vi "TL_init.vi"(0 "Channel #":i32, 1 "TL array":dbl[][](array[numeric]), 3 "Queue cluser":T1, 5 "Mosaic cluster":cluster{dbl[], dbl[]}[](array[cluster]), 7 "N ROIs":i32, 9 "error in":errorcluster, 11 "Start acquisition":bool, 12 "XYGraph":refnum<vi>, 14 "Dt (s)":i32) -> (6 "Ready":bool, 15 "error out":errorcluster)   [LabVIEW 2015]
uses:
  CONTROLS/Q_DAQ_element.ctl
  CONTROLS/Q_camera_element.ctl
  CONTROLS/Q_ASI_stage_element.ctl
  CONTROLS/Q_MCL_piezo_element.ctl
  GLOBAL/Global_DAQ.vi
  GLOBAL/Global_ASI_stage.vi
  GLOBAL/Global_MCL_piezo.vi
  GLOBAL/Global_CAMERA.vi
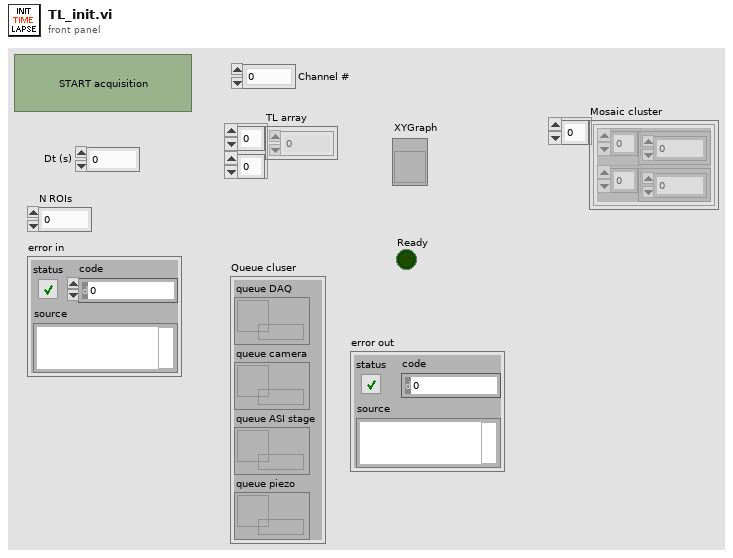
[diagram p1: front panel]
types:
  T1 = cluster{"queue DAQ":refnum<queue>, "queue camera":refnum<queue>, "queue ASI stage":refnum<queue>, "queue piezo":refnum<queue>}
  T2 = cluster{"TL array":dbl[], "XYGraph":refnum<vi>, "Mosaic cluster":cluster{dbl[], dbl[]}[]}
  T3 = typedef "Q_camera_element.ctl" = cluster{"variant":variant, "Instruction":enum16{"CAMERA_idle", "CAMERA_initialize", "CAMERA_error", "CAMERA_security_stop", "CAMERA_not_acquiring", "CAMERA_acquiring", "CAMERA_start_acquiring", "CAMERA_stop_acquiring", "CAMERA_change_exposure", "CAMERA_define_ROI", "CAMERA_cooler", "CAMERA_acquire_movie", "CAMERA_init_scan", "CAMERA_check_new_scan_image", "CAMERA_close_scan", "CAMERA_init_merFISH", "CAMERA_start_acquiring_merFISH", "CAMERA_close_scan_merFISH", "CAMERA_close_merFISH", "CAMERA_init_TL", "CAMERA_start_acquiring_TL", "CAMERA_stop_acquiring_TL", "CAMERA_close_TL", "CAMERA_STOP"}}
  T4 = typedef "Q_MCL_piezo_element.ctl" = cluster{"variant":variant, "Instruction":enum16{"Piezo_idle", "Piezo_initialize", "Piezo_error", "Piezo_security_stop", "Piezo_read_z", "Piezo_move_z", "Piezo_keyboard_move", "Piezo_close_autofocus_calibration_ramp", "Piezo_change_init_state", "Piezo_init_autofocus", "Piezo_init_autofocus_merFISH_TL", "Piezo_autofocus", "Piezo_autofocus_merFISH_TL", "Piezo_stop_autofocus", "Piezo_stop_autofocus_merFISH_TL", "Piezo_autofocus_lost", "Piezo_resume_autofocus_merFISH_TL", "Piezo_check_z_position_merFISH_TL", "Piezo_init_ramp", "Piezo_move_z_ramp", "Piezo_close_ramp", "Piezo_close_merFISH", "Piezo_init_TL", "Piezo_close_ramp_TL", "Piezo_close_TL", "Piezo_stop"}}
  T5 = typedef "Q_DAQ_element.ctl" = cluster{"variant":variant, "Instruction":enum16{"DAQ_idle", "DAQ_initialize", "DAQ_error", "DAQ_security_stop", "DAQ_start_QPD", "DAQ_change_QPD_display", "DAQ_read_display_QPD_signal", "DAQ_QPD_init_autofocus", "DAQ_read_display_send_QPD_signal", "DAQ_close_autofocus_calibration_ramp", "DAQ_close_autofocus", "DAQ_405", "DAQ_488", "DAQ_561", "DAQ_641", "DAQ_zero_all", "DAQ_init_single_scan", "DAQ_single_scan", "DAQ_two_way_valve", "DAQ_init_merFISH", "DAQ_scan_merFISH", "DAQ_photobleaching_merFISH", "DAQ_close_merFISH", "DAQ_init_TL", "DAQ_synchro_TL", "DAQ_close_task_TL", "DAQ_close_TL", "DAQ_stop"}}
  T6 = typedef "Q_ASI_stage_element.ctl" = cluster{"variant":variant, "Instruction":enum16{"ASI_idle", "ASI_initialize", "ASI_error", "ASI_security_stop", "ASI_read_XYZ", "ASI_up", "ASI_down", "ASI_left", "ASI_right", "ASI_save_XY", "ASI_move_to_XY", "ASI_brightfield", "ASI_init_scan", "ASI_init_merFISH", "ASI_move_to_XY_merFISH", "ASI_move_to_Z_merFISH", "ASI_init_autofocus_search_merFISH", "ASI_close_autofocus_search_merFISH", "ASI_adjust_piezo_autofocus_merFISH", "ASI_set_piezo_autofocus_to_reference_position_merFISH_TL", "ASI_close_merFISH", "ASI_init_TL", "ASI_move_mosaic_TL", "ASI_brightfield_TL", "ASI_close_TL", "ASI_stop"}}
  T7 = enum16{"DAQ_idle", "DAQ_initialize", "DAQ_error", "DAQ_security_stop", "DAQ_start_QPD", "DAQ_change_QPD_display", "DAQ_read_display_QPD_signal", "DAQ_QPD_init_autofocus", "DAQ_read_display_send_QPD_signal", "DAQ_close_autofocus_calibration_ramp", "DAQ_close_autofocus", "DAQ_405", "DAQ_488", "DAQ_561", "DAQ_641", "DAQ_zero_all", "DAQ_init_single_scan", "DAQ_single_scan", "DAQ_two_way_valve", "DAQ_init_merFISH", "DAQ_scan_merFISH", "DAQ_photobleaching_merFISH", "DAQ_close_merFISH", "DAQ_init_TL", "DAQ_synchro_TL", "DAQ_close_task_TL", "DAQ_close_TL", "DAQ_stop"}
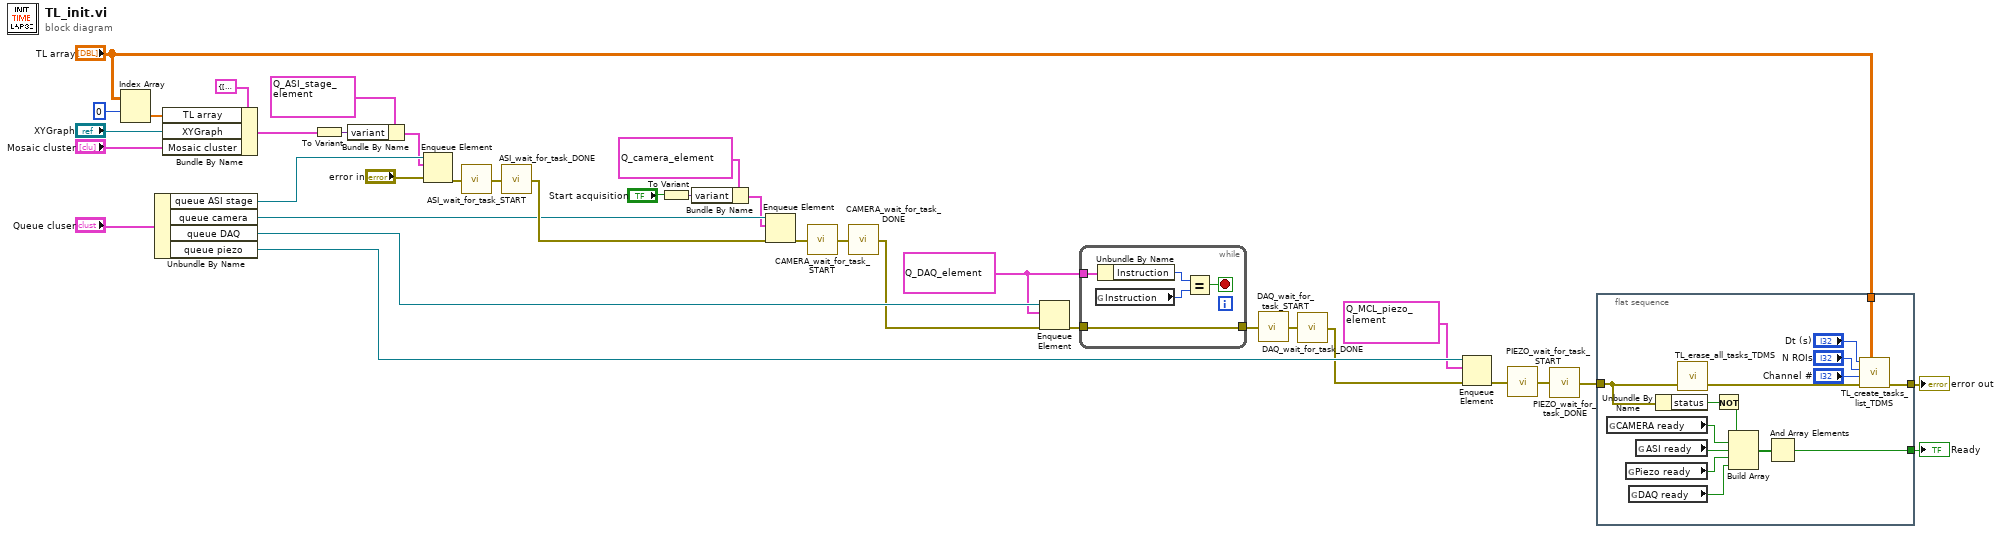
[diagram p0: block diagram]
diagram:
  w8 = T5 {"variant"=variant, "Instruction"=enum."DAQ_init_TL"} ("element")
  n1 = Index Array(array="TL array", index (row)=0) -> (element=w3:dbl[])  [unwired: 1 in]
  n2 = Unbundle By Name("Queue cluser") -> ("queue ASI stage"=w30:refnum<queue>, "queue camera"=w29:refnum<queue>, "queue DAQ"=w28:refnum<queue>, "queue piezo"=w25:refnum<queue>)
  n3 = Bundle By Name(cluster=T2 {"TL array"=[], "XYGraph"=refnum, "Mosaic cluster"=[]}, "TL array"=w3, "XYGraph"="XYGraph", "Mosaic cluster"="Mosaic cluster") -> (w4:T2)
  n4 = To Variant(anything=w4) -> (Variant=w16:variant)
  n5 = Bundle By Name(cluster=T6 {"variant"=variant, "Instruction"=enum."ASI_init_TL"} ("element"), "variant"=w16) -> (w17:T6)
  n6 = Enqueue Element(queue=w30, element=w17, error in (no error)="error in") -> (error out=w35:errorcluster)  [unwired: 1 in, 2 out]
  n7 = call "ASI_wait_for_task_START.vi"("error in"=w35) -> ("error out"=w36:errorcluster)
  n8 = call "ASI_wait_for_task_DONE.vi"("error in"=w36) -> ("error out"=w37:errorcluster)
  n9 = To Variant(anything="Start acquisition") -> (Variant=w12:variant)
  n10 = Bundle By Name(cluster=T3 {"variant"=variant, "Instruction"=enum."CAMERA_init_TL"} ("Q_ANDOR_element"), "variant"=w12) -> (w13:T3)
  n11 = Enqueue Element(queue=w29, element=w13, error in (no error)=w37) -> (error out=w33:errorcluster)  [unwired: 1 in, 2 out]
  n12 = call "CAMERA_wait_for_task_START.vi"("error in"=w33) -> ("error out"=w34:errorcluster)
  n13 = call "CAMERA_wait_for_task_DONE.vi"("error in"=w34) -> ("error out"=w27:errorcluster)
  n14 = Enqueue Element(queue=w28, element=w8, error in (no error)=w27) -> (error out=w10:errorcluster)  [unwired: 1 in, 2 out]
  n15 = while {
    tunnel: w10 -> [w39]
    tunnel: [w39] -> w9
    tunnel: w8 -> [w38]
    stop <- w41 stop-if-true
    n16 = global read "Global_DAQ.vi" "Instruction"() -> (w42:T7)
    n17 = Unbundle By Name(w38) -> ("Instruction"=w40:T7)
    n18 = Equal?(x=w40, y=w42) -> (x = y?=w41:bool)
  }
  n19 = call "DAQ_wait_for_task_START.vi"("error in"=w9) -> ("error out"=w26:errorcluster)
  n20 = call "DAQ_wait_for_task_DONE.vi"("error in"=w26) -> ("error out"=w24:errorcluster)
  n21 = Enqueue Element(queue=w25, element=T4 {"variant"=variant, "Instruction"=enum."Piezo_init_TL"}, error in (no error)=w24) -> (error out=w21:errorcluster)  [unwired: 1 in, 2 out]
  n22 = call "PIEZO_wait_for_task_START.vi"("error in"=w21) -> ("error out"=w20:errorcluster)
  n23 = call "PIEZO_wait_for_task_DONE.vi"("error in"=w20) -> ("error out"=w19:errorcluster)
  n24 = flat-sequence {
    tunnel: [w52] -> w23
    tunnel: w19 -> [w49]
    tunnel: [w48] -> w22
    tunnel: "TL array" -> [w43]
    frame #0 {
      n25 = global read "Global_CAMERA.vi" "CAMERA ready"() -> (w55:bool)
      n26 = global read "Global_MCL_piezo.vi" "Piezo ready"() -> (w56:bool)
      n27 = global read "Global_DAQ.vi" "DAQ ready"() -> (w53:bool)
      n28 = global read "Global_ASI_stage.vi" "ASI ready"() -> (w57:bool)
      n29 = Unbundle By Name(w49) -> ("status"=w50:bool)
      n30 = call "TL_erase_all_tasks_TDMS.vi"("error in"=w49) -> ("error out"=w45:errorcluster)  [unwired: 2 in]
      n31 = Not(x=w50) -> (.not. x?=w51:bool)
      n32 = Build Array(w51, w55, w57, w56, w53) -> (w54:bool[])
      n33 = And Array Elements(Boolean array=w54) -> (logical AND=w52:bool)
      n34 = call "TL_create_tasks_list_TDMS.vi"("TL array"=w43, "error in"=w45, "Channel #"="Channel #", "N ROIs"="N ROIs", "Dt (s)"="Dt (s)") -> ("error out"=w48:errorcluster)  [unwired: 3 in]
    }
  }
  "error out" <- w22
  "Ready" <- w23
